vi "Split and Merge Filter.vi"(10 "Threshold":dbl, 11 "output cluster":cluster{dbl[], dbl[]}) -> (2 "Array":cluster{dbl[], dbl[]}[](array[cluster]))   [LabVIEW 2017]
uses:
  <vilib>/Analysis/NI_AALPro.lvlib
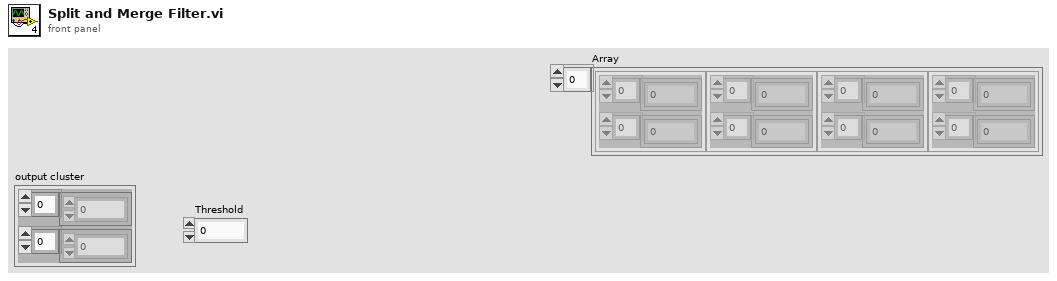
[diagram p1: front panel]
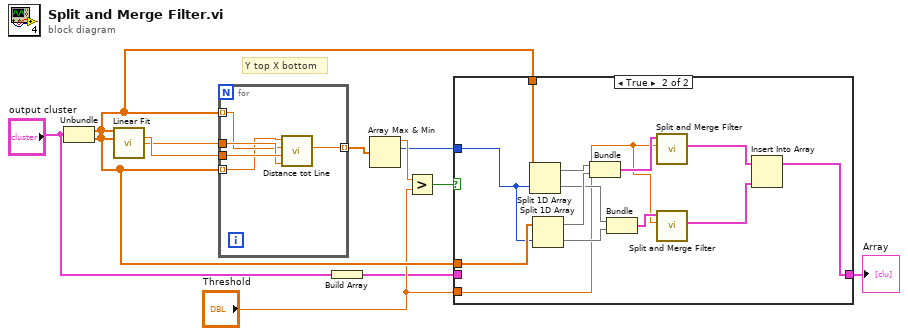
[diagram p0: block diagram]
diagram:
  # "Y top X bottom"
  n1 = Unbundle("output cluster") -> (w7:dbl[], w6:dbl[])
  n2 = call <vilib>:"Linear Fit.vi"("Y"=w7, "X"=w6) -> ("slope"=w12:dbl, "intercept"=w11:dbl)  [unwired: 9 in, 3 out]
  n3 = for {
    tunnel: w7 -> [w15] mode=indexing
    tunnel: w6 -> [w14] mode=indexing
    tunnel: w12 -> [w17]
    tunnel: w11 -> [w16]
    tunnel: [w13] -> w10 mode=indexing
    n4 = call "Distance tot Line.vi"("B"=w16, "M"=w17, "Y"=w15, "X"=w14) -> ("Distance"=w13:dbl)  [unwired: 7 in]
  }
  n5 = Build Array("output cluster") -> (w2:cluster{dbl[], dbl[]}[])
  n6 = Array Max & Min(array=w10) -> (max value=w8:dbl, max index (indices)=w5:i32)  [unwired: 2 out]
  n7 = Greater?(x=w8, y="Threshold") -> (0:w9:bool)
  n8 = case shown="True" w9 {
    tunnel: w7 -> [_ w31]
    tunnel: w6 -> [_ w30]
    tunnel: w5 -> [_ w29]
    tunnel: "Threshold" -> [_ w22]
    tunnel: w2 -> [w18 _]
    tunnel: [w18 w19] -> w1
    frame False {
    }
    frame True {
      n9 = Split 1D Array(array=w31, index=w29) -> (first subarray=w28:dbl[], second subarray=w25:dbl[])
      n10 = Split 1D Array(array=w30, index=w29) -> (first subarray=w27:dbl[], second subarray=w24:dbl[])
      n11 = Bundle(w28, w27) -> (w26:cluster{dbl[], dbl[]})  [unwired: 1 in]
      n12 = Bundle(w25, w24) -> (w23:cluster{dbl[], dbl[]})  [unwired: 1 in]
      n13 = call "Split and Merge Filter.vi"("Threshold"=w22, "output cluster"=w26) -> ("Array"=w21:cluster{dbl[], dbl[]}[])  [unwired: 9 in]
      n14 = call "Split and Merge Filter.vi"("Threshold"=w22, "output cluster"=w23) -> ("Array"=w20:cluster{dbl[], dbl[]}[])  [unwired: 9 in]
      n15 = Insert Into Array(array=w21, new element=w20) -> (w19:cluster{dbl[], dbl[]}[])  [unwired: 1 in]
    }
  }
  "Array" <- w1
